vi "Read Access Scope.vi"(8 "error in (no error)":errorcluster, 11 "Vi in":refnum<class "Vi.lvclass">) -> (0 "error out":errorcluster, 2 "Access Scope":T1(ring), 3 "Vi out":refnum<class "Vi.lvclass">)   [LabVIEW 2021, in "TAF Proj Document Type.lvlib" / "Vi.lvclass"]
uses:
  <vilib>/Wovalab/AntiDoc/Document Type/Add-ons/LabVIEW TAF Project/Vi/Vi.lvclass
  <vilib>/Wovalab/AntiDoc/Document Type/Add-ons/LabVIEW TAF Project/Vi/Vi.lvclass/Vi.ctl
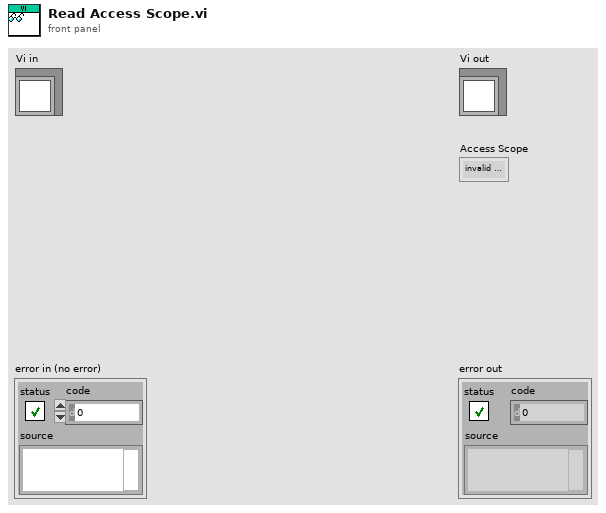
[diagram p1: front panel]
types:
  T1 = enum32{"invalid scope", "public", "private", "protected", "community"}
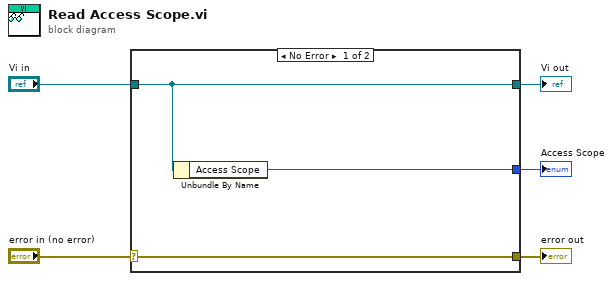
[diagram p0: block diagram]
diagram:
  n1 = case shown="No Error" "error in (no error)" {
    selector: "error in (no error)" -> [w8 w9]
    tunnel: [w8 w9] -> w4
    tunnel: [w7 w10] -> w2
    tunnel: "Vi in" -> [w7 w10]
    tunnel: [w6 _] -> w1
    frame No Error {
      n2 = Unbundle By Name(w7) -> ("Access Scope"=w6:T1)
    }
    frame Error {
    }
  }
  "error out" <- w4
  "Vi out" <- w2
  "Access Scope" <- w1
